vi "clear all subscription.vi"(8 "error in":errorcluster, 11 "refnum in":T1) -> (0 "error out":errorcluster, 3 "refnum in":T1)   [LabVIEW 2020, in "Publisher Subscriber.lvlib"]
uses:
  Publisher Subscriber.lvlib
  Controls/node refnum.ctl
  Controls/node dvr data.ctl
  Controls/data cluster.ctl
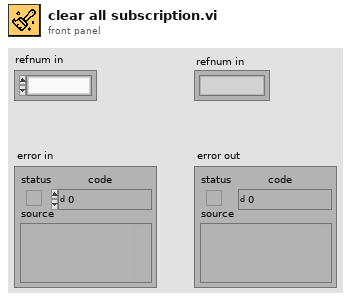
[diagram p1: front panel]
types:
  T1 = typedef "Publisher Subscriber.lvlib/node refnum.ctl" = refnum<k1>
  T2 = typedef "Publisher Subscriber.lvlib/node dvr data.ctl" = cluster{"queue ref":refnum<queue>, "subscription map ref":refnum<data-value>, "Command":string, "Data":variant, "Subscriptions []":set{string}, "variable dvr refs":refnum<data-value>}
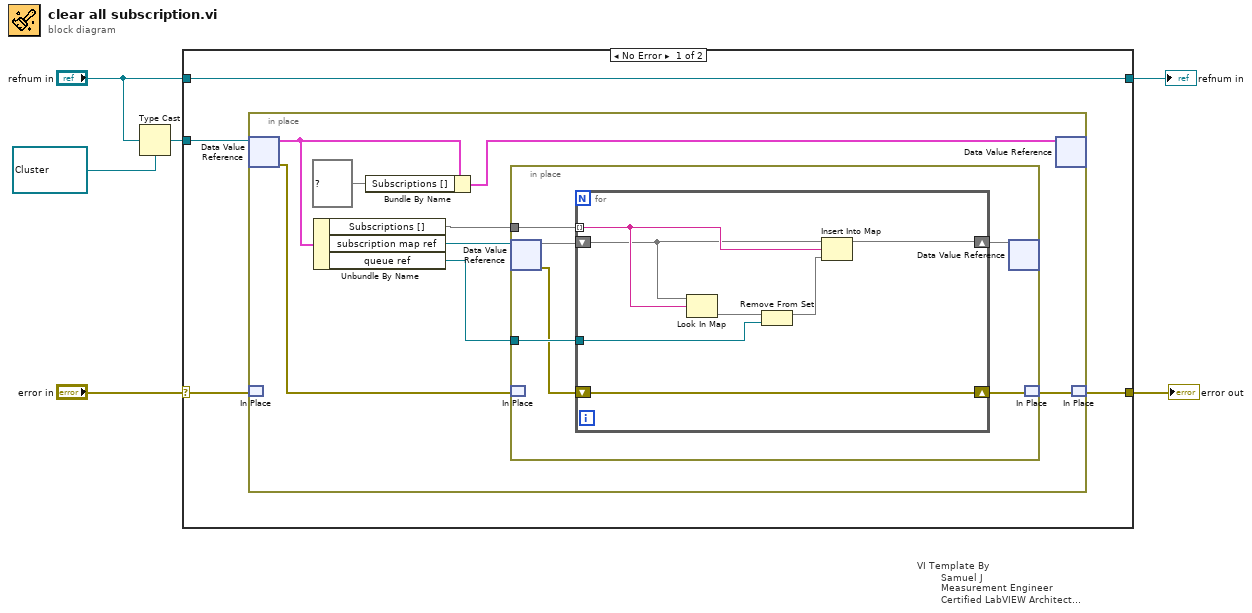
[diagram p0: block diagram]
diagram:
  n1 = Type Cast(type=refnum<data-value> refnum ("data value reference"), x="refnum in") -> (*(type *) &x=w3:refnum<data-value>)
  n2 = case "VI Template By\n        Samuel J\n        Measurement Engineer\n        Certified LabVIEW Architect\n        Vestas Technology R&D Chennai" shown="No Error" "error in" {
    selector: "error in" -> [w8 w33]
    tunnel: [w7 w33] -> w5
    tunnel: w3 -> [w9 _]
    tunnel: [w10 w32] -> w2
    tunnel: "refnum in" -> [w10 w32]
    frame No Error {
      n3 = in-place {
        n4 = in-place-dvr #1(w9) -> (w18:T2, w12:errorcluster)
        n5 = in-place-match #2(w8) -> ()  [unwired: 1 out]
        n6 = Unbundle By Name(w18) -> ("Subscriptions []"=w14:set{string}, "subscription map ref"=w15:refnum<data-value>, "queue ref"=w13:refnum<queue>)
        n7 = Bundle By Name(cluster=w18, "Subscriptions []"=set{string} {}) -> (w17:T2)
        n8 = in-place {
          in-place-border: w14 -> [w22]
          in-place-border: w13 -> [w21]
          n9 = in-place-dvr #3(w15) -> (w24:map{string, set{refnum<queue>}}, w19:errorcluster)
          n10 = in-place-match #4(w12) -> ()  [unwired: 1 out]
          n11 = for {
            shift-right: [w29] -> w23
            shift-left: w24 -> [w30]
            tunnel: w22 -> [w31] mode=indexing
            shift-right: [w26] -> w20
            shift-left: w19 -> [w26]
            tunnel: w21 -> [w27]
            n12 = Look In Map(map=w30, key=w31) -> (value=w28:set{refnum<queue>})  [unwired: 1 in, 1 out]
            n13 = Remove From Set(10:w27, 11:w28) -> (3:w25:set{refnum<queue>})  [unwired: 1 out]
            n14 = Insert Into Map(map in=w30, key=w31, value=w25) -> (map out=w29:map{string, set{refnum<queue>}})  [unwired: 2 out]
          }
          n15 = in-place-dvr #3(w23) -> ()  [unwired: 2 out]
          n16 = in-place-match #4(w20) -> (w11:errorcluster)
        }
        n17 = in-place-dvr #1(w17) -> ()  [unwired: 2 out]
        n18 = in-place-match #2(w11) -> (w7:errorcluster)
      }
    }
    frame Error {
    }
  }
  "error out" <- w5
  "refnum in" <- w2
